vi "Conf Count.vi"(8 "error in (no error)":errorcluster, 11 "IncCounter":T1) -> (0 "error out":errorcluster, 3 "IncCounter Out":T1)   [LabVIEW 2014, in "MSX-E3711_dll.lvlib"]
uses:
  MSX-E3711_dll.lvlib
panel:
  in  "Reducción":sgl
  in  "Cantidad de Pulsos":sgl
  in  "Cancelar":bool
  in  "Save Button":bool
  # "Configurar Encoder"
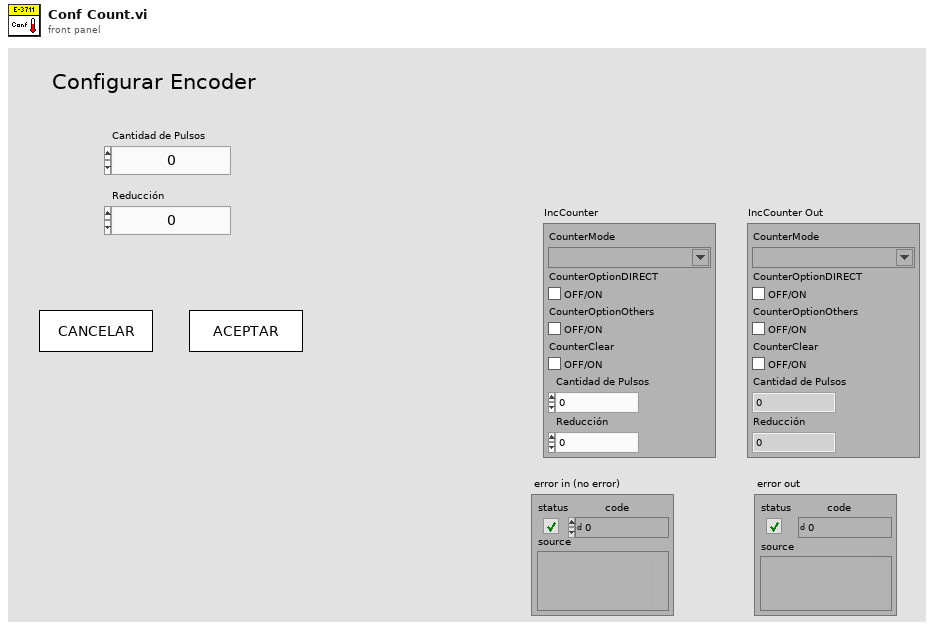
[diagram p1: front panel]
types:
  T1 = cluster{"CounterMode":string, "CounterOptionDIRECT  ":bool, "CounterOptionOthers":bool, "CounterClear ":bool, "Cantidad de Pulsos":sgl, "Reducción":sgl}
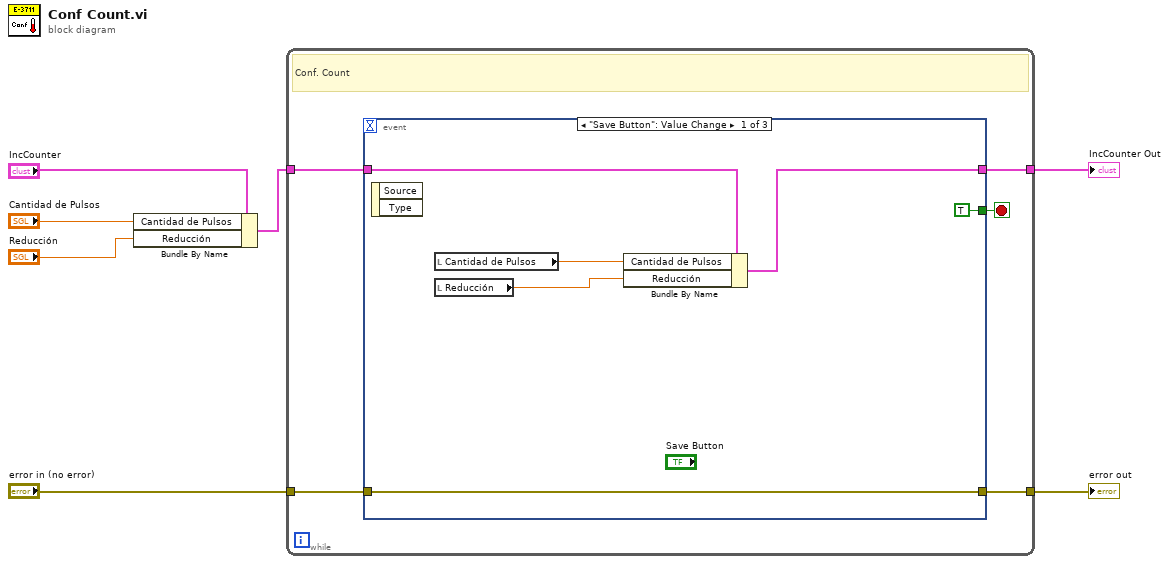
[diagram p0: block diagram]
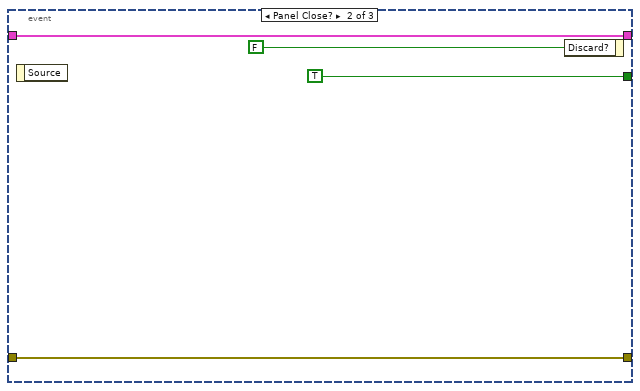
[diagram p2: hidden frame]
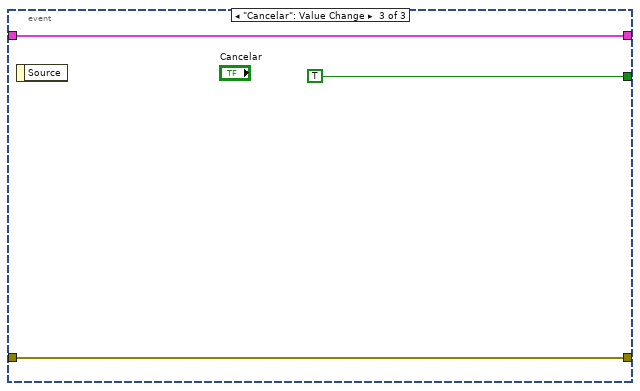
[diagram p3: hidden frame]
diagram:
  n1 = Bundle By Name(cluster="IncCounter", "Cantidad de Pulsos"="Cantidad de Pulsos", "Reducción"="Reducción") -> (w5:T1)
  n2 = while {
    tunnel: [w11] -> w4
    tunnel: w5 -> [w10]
    tunnel: "error in (no error)" -> [w9]
    tunnel: [w8] -> w6
    stop <- w12 stop-if-true
    # "Conf. Count"
    n3 = event shown="[0] \"Save Button\": Value Change" {
      selector: _ -> [_ _ _]
      dyn-events: _ -> [_ _ _]
      timeout: _ -> [_ _ _]
      tunnel: [TRUE ("Save Button") TRUE ("Save Button") TRUE ("Save Button")] -> w12
      tunnel: [w15 w20 w24] -> w11
      tunnel: w10 -> [w16 w20 w24]
      tunnel: w9 -> [w17 w19 w23]
      tunnel: [w17 w19 w23] -> w8
      event "Save Button": Value Change {
        n4 = event-data() -> ()  [unwired: 1 in, 2 out]
        n5 = local read "Cantidad de Pulsos"() -> (w14:sgl)
        n6 = local read "Reducción"() -> (w13:sgl)
        n7 = Bundle By Name(cluster=w16, "Cantidad de Pulsos"=w14, "Reducción"=w13) -> (w15:T1)
      }
      event Panel Close? {
        n8 = event-data() -> ()  [unwired: 1 in, 1 out]
        n9 = event-data("Discard?"=FALSE) -> ()  [unwired: 1 in, 1 out]
      }
      event "Cancelar": Value Change {
        n10 = event-data() -> ()  [unwired: 1 in, 1 out]
      }
    }
  }
  "error out" <- w6
  "IncCounter Out" <- w4
